vi "lsl create outlet.vi"(8 "error in (no error)":errorcluster, 9 "max_buffered":i32=360, 10 "chunk_size":i32, 11 "streaminfo":T2) -> (0 "error out":errorcluster, 3 "outlet":T1)   [LabVIEW 2018, in "liblsl-LabVIEW.lvlib"]
doc: "extern LIBLSL_C_API lsl_outlet lsl_create_outlet(lsl_streaminfo info, int32_t chunk_size, int32_t max_buffered);"
uses:
  <userlib>/liblsl-LabVIEW/liblsl-LabVIEW.lvlib
  <userlib>/liblsl-LabVIEW/Custom Controls/lsl_streaminfo.ctl
  <userlib>/liblsl-LabVIEW/Custom Controls/lsl_outlet.ctl
  <userlib>/liblsl-LabVIEW/liblsl64.dll
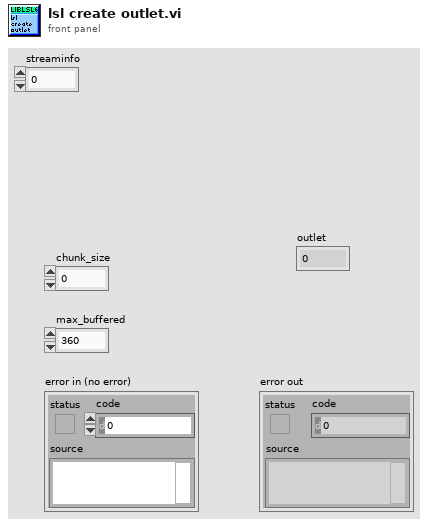
[diagram p1: front panel]
types:
  T1 = typedef "liblsl-LabVIEW.lvlib/lsl_outlet.ctl" = u64
  T2 = typedef "liblsl-LabVIEW.lvlib/lsl_streaminfo.ctl" = u64
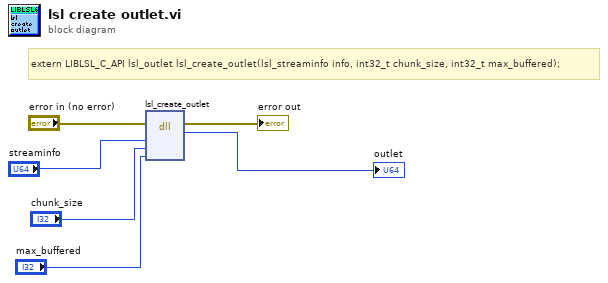
[diagram p0: block diagram]
diagram:
  # "extern LIBLSL_C_API lsl_outlet lsl_create_outlet(lsl_streaminfo info, int32_t chunk_size, int32_t max_buffered);"
  n1 = dll-call lib="C:/Program Files/National Instruments/LabVIEW 2018/user.lib/liblsl-LabVIEW/liblsl64.dll" fn="lsl_create_outlet"(error in="error in (no error)", "info"="streaminfo", "chunk_size"="chunk_size", "max_buffered"="max_buffered") -> (error out=→"error out":errorcluster, "return type"=→"outlet":u64)  [unwired: 5 in, 1 out]
